vi "SaveSettingToFile.vi"(8 "error in (no error)":errorcluster, 11 "ProgramSettings in":refnum<class "ProgramSettings.lvclass">) -> (0 "error out":errorcluster, 3 "ProgramSettings out":refnum<class "ProgramSettings.lvclass">)   [LabVIEW 2019, in "ProgramSettings.lvclass"]
uses:
  ProgramSettings.lvclass
  ProgramSettings.lvclass/ProgramSettings.ctl
  <vilib>/Utility/xml.llb/Write to XML File(string).vi
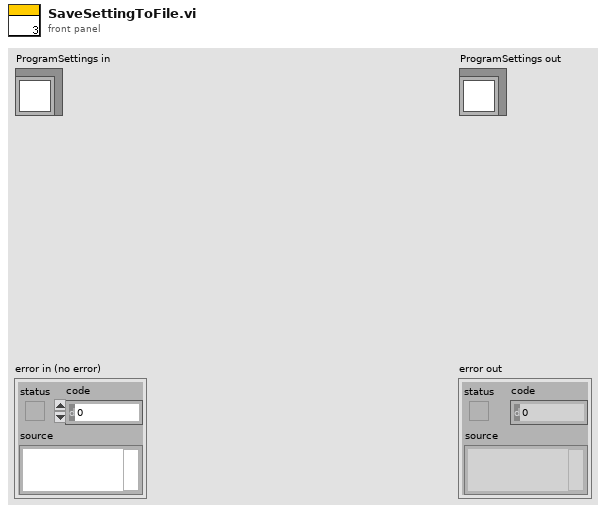
[diagram p1: front panel]
types:
  T1 = cluster{"Serial Port for strømforsyning":refnum<visa-resource-name>}
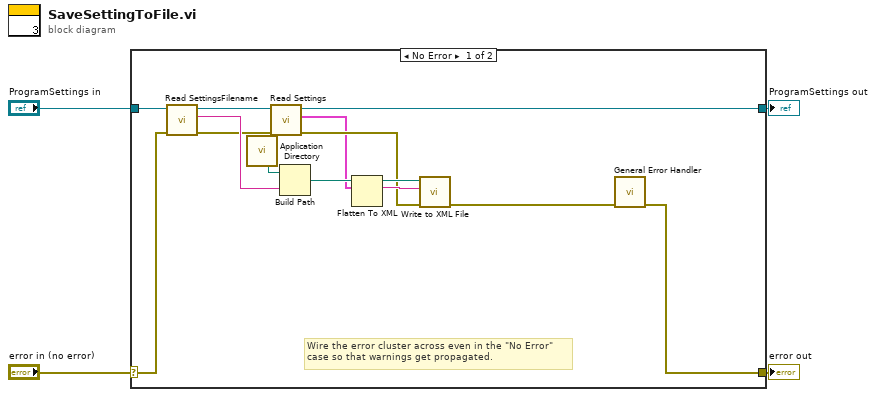
[diagram p0: block diagram]
diagram:
  n1 = case shown="No Error" "error in (no error)" {
    selector: "error in (no error)" -> [w13 w19]
    tunnel: [w11 w19] -> w3
    tunnel: [w9 w18] -> w1
    tunnel: "ProgramSettings in" -> [w14 w18]
    frame No Error {
      # "Wire the error cluster across even in the \"No Error\"\ncase so that warnings get propagated."
      n2 = call "Read SettingsFilename.vi"("error in (no error)"=w13, "ProgramSettings in"=w14) -> ("error out"=w8:errorcluster, "SettingsFilename"=w17:string, "ProgramSettings out"=w10:refnum<class "ProgramSettings.lvclass">)  [unwired: 7 in]
      n3 = call <vilib>:"Application Directory.vi"() -> ("Application Directory"=w5:path)
      n4 = call "Read Settings.vi"("error in (no error)"=w8, "ProgramSettings in"=w10) -> ("error out"=w7:errorcluster, "Settings"=w6:T1, "ProgramSettings out"=w9:refnum<class "ProgramSettings.lvclass">)  [unwired: 7 in]
      n5 = Build Path(base path=w5, name or relative path=w17) -> (appended path=w16:path)
      n6 = Flatten To XML(anything=w6) -> (xml string=w15:string)
      n7 = call-poly <vilib>:"Write to XML File.vi"("error in (no error)"=w7, "XML Input"=w15, "XML File Path"=w16) -> ("error out"=w12:errorcluster)  [unwired: 6 in, 2 out]
      n8 = call <vilib>:"General Error Handler.vi"("error in (no error)"=w12) -> ("error out"=w11:errorcluster)  [unwired: 10 in, 4 out]
    }
    frame Error {
    }
  }
  "error out" <- w3
  "ProgramSettings out" <- w1
